vi "ErrorHandler.vi"(0 "Additional Information":string, 11 "error in (no error)":errorcluster) -> (15 "error out":errorcluster)   [LabVIEW 2016]
uses:
  <vilib>/Utility/error.llb/DialogType.ctl
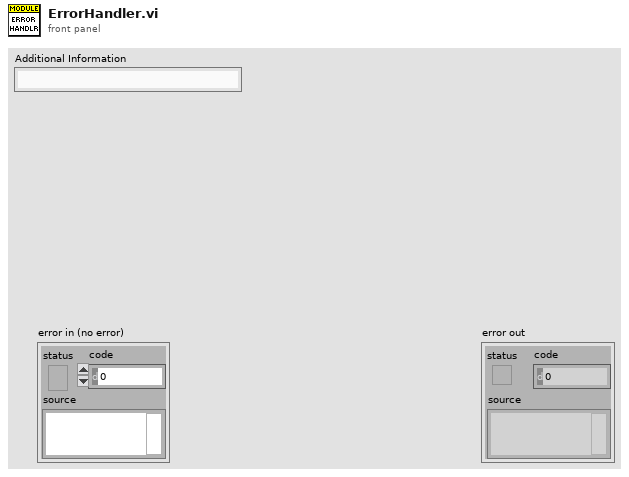
[diagram p1: front panel]
types:
  T1 = enum16{"open", "replace", "create", "open or create", "replace or create", "replace or create with confirmation"}
  T2 = typedef "DialogType.ctl" = u16
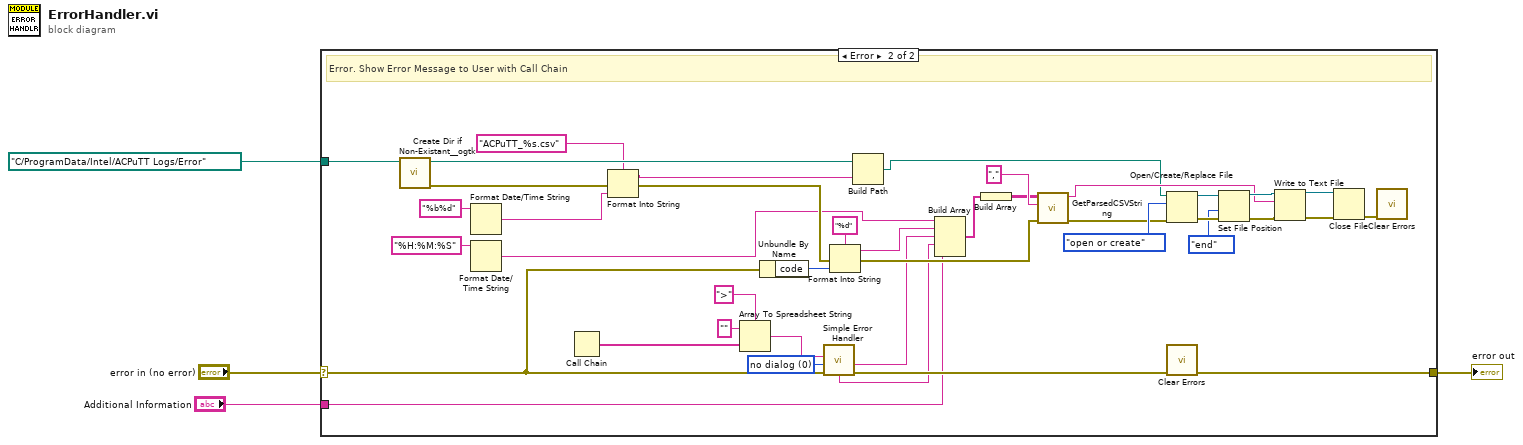
[diagram p0: block diagram]
diagram:
  n1 = case shown="Error" "error in (no error)" {
    selector: "error in (no error)" -> [w5 w22]
    tunnel: [w5 w8] -> w3
    tunnel: "Additional Information" -> [_ w6]
    tunnel: path "C:/ProgramData/Intel/ACPuTT Logs/Error" ("Directory Path") -> [_ w17]
    frame No Error {
      # "Wire the error cluster across even in the \"No Error\"\ncase so that warnings get propagated."
    }
    frame Error {
      w41 = T2 0 items=["no dialog", "OK message", "continue or stop message", "OK message + warnings", "continue/stop + warnings"] ("type of dialog (OK msg:1)")
      # "Error. Show Error Message to User with Call Chain"
      n2 = call "Create Dir if Non-Existant__ogtk.vi"("Directory Path"=w17) -> ("error out"=w20:errorcluster, "dup Directory Path"=w18:path)  [unwired: 8 in, 1 out]
      n3 = Format Date/Time String(time format string (%c)="%b%d") -> (date/time string=w11:string)  [unwired: 2 in]
      n4 = Format Date/Time String(time format string (%c)="%H:%M:%S") -> (date/time string=w10:string)  [unwired: 2 in]
      n5 = Call Chain() -> (call chain=w45:string[])
      n6 = Format Into String(format string="ACPuTT_%s.csv", error in=w20, w11) -> (resulting string=w13:string, error out=w15:errorcluster)  [unwired: 1 in]
      n7 = Array To Spreadsheet String(delimiter (Tab)=">", array=w45, 3:"" ("format string")) -> (spreadsheet string=w43:string)
      n8 = Unbundle By Name(w22) -> ("code"=w39:i32)
      n9 = call <vilib>:"Simple Error Handler.vi"("error source (\" \")"=w43, "type of dialog (OK msg:1)"=w41, "error in (no error)"=w22) -> ("source out"=w21:string, "error out"=w42:errorcluster, "message"=w7:string)  [unwired: 2 in, 2 out]
      n10 = Format Into String(format string="%d", error in=w15, w39) -> (resulting string=w38:string, error out=w37:errorcluster)  [unwired: 1 in]
      n11 = Build Path(base path=w18, name or relative path=w13) -> (appended path=w16:path)
      n12 = Build Array(w10, w38, w21, w7, w6) -> (w35:string[])
      n13 = Build Array(w35) -> (w34:string[][])
      n14 = call "GetParsedCSVString.vi"("error in (no error)"=w37, "Delimiter"=",", "Info to write"=w34) -> ("error out"=w26:errorcluster, "CSVStringOut"=w23:string)  [unwired: 7 in]
      n15 = Open/Create/Replace File(file path (use dialog)=w16, error in=w26, operation (0:open)=T1."open or create") -> (refnum out=w28:refnum<file>, error out=w29:errorcluster)  [unwired: 3 in, 1 out]
      n16 = call <vilib>:"Clear Errors.vi"("error in (no error)"=w42) -> ("error out"=w8:errorcluster)  [unwired: 5 in, 1 out]
      n17 = Set File Position(refnum=w28, from (0:start)=enum16{"start", "end", "current"}."end", error in=w29) -> (refnum out=w24:refnum<file>, error out=w25:errorcluster)  [unwired: 1 in]
      n18 = Write to Text File(file (use dialog)=w24, text=w23, error in=w25) -> (refnum out=w32:refnum<file>, error out=w33:errorcluster)  [unwired: 1 in, 1 out]
      n19 = Close File(refnum=w32, error in=w33) -> (error out=w31:errorcluster)  [unwired: 1 out]
      n20 = call <vilib>:"Clear Errors.vi"("error in (no error)"=w31) -> ()  [unwired: 5 in, 2 out]
    }
  }
  "error out" <- w3
